vi "Setup.vi"(8 "error in (no error)":errorcluster, 11 "LUnit My Test In":refnum<class "My Test.lvclass">) -> (0 "error out":errorcluster, 3 "LUnit My Test Out":refnum<class "My Test.lvclass">)   [LabVIEW 2020, in "My Test.lvclass"]
doc: "Setup method called by the testing framework to set up test fixture before each test method is called."
uses:
  My Test.lvclass
  My Test.lvclass/My Test.ctl
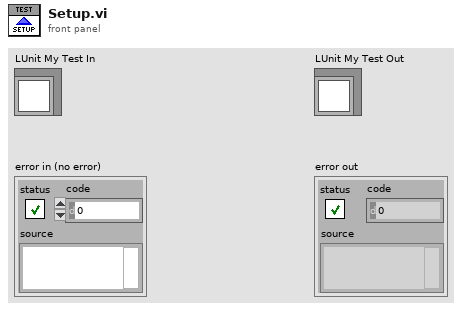
[diagram p1: front panel]
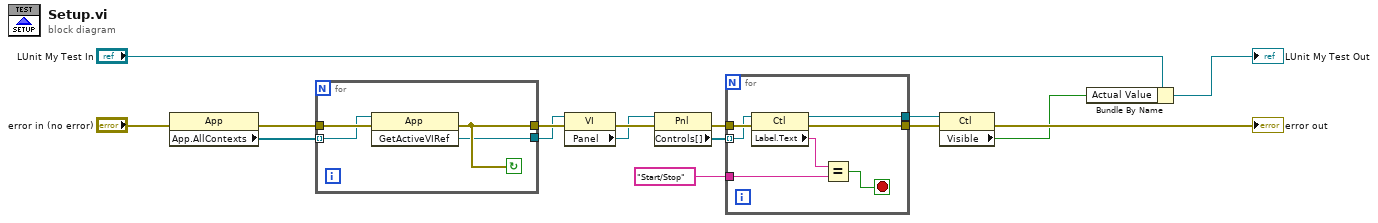
[diagram p0: block diagram]
diagram:
  n1 = property class="App"(error in="error in (no error)") -> (error out=w15:errorcluster, "App.AllContexts"=w12:refnum<vi>[])  [unwired: 1 in, 1 out]
  n2 = for {
    tunnel: [w18] -> w11
    tunnel: w12 -> [w19] mode=indexing
    tunnel: w15 -> [w20]
    tunnel: [w17] -> w10
    stop <- w18 continue-if-true
    n3 = invoke class="App" method="GetActiveVIRef"(reference=w19, error in=w20) -> (error out=w18:errorcluster, "GetActiveVIRef"=w17:refnum<vi>)  [unwired: 1 in, 1 out]
  }
  n4 = property class="VI"(reference=w10, error in=w11) -> (error out=w9:errorcluster, "Panel"=w6:refnum<vi>)  [unwired: 1 out]
  n5 = property class="Pnl"(reference=w6, error in=w9) -> (error out=w8:errorcluster, "Controls[]"=w5:refnum<vi>[])  [unwired: 1 out]
  n6 = for {
    tunnel: w8 -> [w27]
    tunnel: w5 -> [w25] mode=indexing
    tunnel: "Start/Stop" ("Control Name") -> [w23]
    tunnel: [w22] -> w3
    tunnel: [w26] -> w7
    stop <- w21 stop-if-true
    n7 = property class="Ctl"(reference=w25, error in=w27) -> (reference out=w22:refnum<vi>, error out=w26:errorcluster, "Label.Text"=w24:string)
    n8 = Equal?(x=w24, y=w23) -> (x = y?=w21:bool)
  }
  n9 = property class="Ctl"(reference=w3, error in=w7) -> (error out=→"error out":errorcluster, "Visible"=w1:bool)  [unwired: 1 out]
  n10 = Bundle By Name(cluster="LUnit My Test In", "Actual Value"=w1) -> (→"LUnit My Test Out":refnum<class "My Test.lvclass">)
